vi "Theil-Sen.vi"(5 "Aligning array sizes? (T)":bool=TRUE, 6 "error in (no error)":errorcluster, 7 "Sen parameter":enum16{"Auto", "On", "Off"}(ring), 8 "input_Y":dbl[](array[numeric]), 9 "input_X":dbl[](array[numeric])) -> (0 "error out":errorcluster, 1 "b":dbl format="%.6g", 2 "m":dbl format="%.6g", 3 "output_Y":dbl[](array[numeric]))   [LabVIEW 2010]
doc: "The Theil–Sen estimator of a set of two-dimensional points (xi, yi) is the median m of the slopes (yj - yi)/(xj - xi) determined by all pairs of sample points. Sen extended this definition to handle the case in which two data points have the same x coordinate. In Sen's definition, one takes the median of the slopes defined only from pairs of points having distinct x coordinates.\nOnce the slope m has been determined, one may determine a line from the sample points by setting the y-intercept b to be the median of the values yi - mxi. The fit line is then the line y = mx + b with coefficients m and b in slope–intercept form."
uses:
  <vilib>/Analysis/NI_AALBase.lvlib
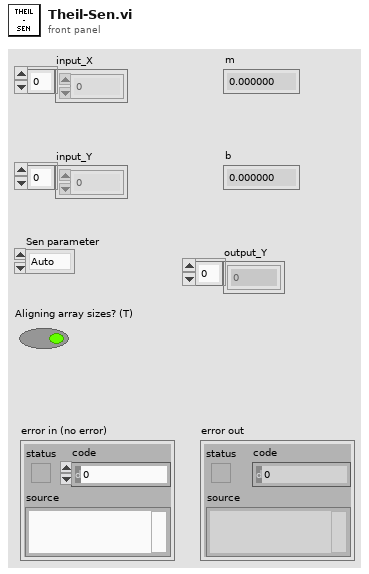
[diagram p1: front panel]
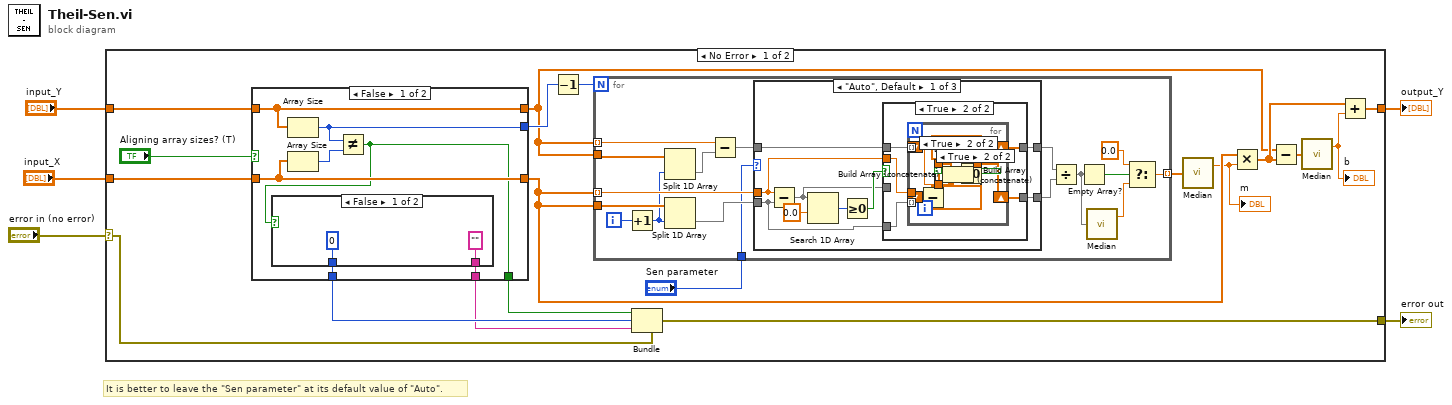
[diagram p0: block diagram]
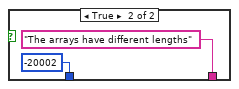
[diagram p2: hidden frame]
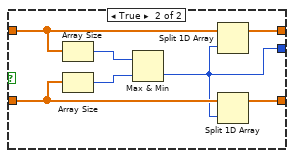
[diagram p3: hidden frame]
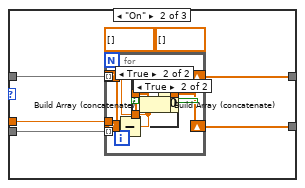
[diagram p7: hidden frame]
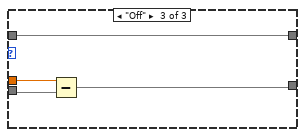
[diagram p10: hidden frame]
diagram:
  # "It is better to leave the \"Sen parameter\" at its default value of \"Auto\"."
  n1 = case shown="No Error" "error in (no error)" {
    selector: "error in (no error)" -> [w10 w124]
    tunnel: "input_X" -> [w24 _]
    tunnel: "input_Y" -> [w22 w123]
    tunnel: [w13 w124] -> w3
    tunnel: [w9 w123] -> w1
    frame No Error {
      n2 = case shown="False" "Aligning array sizes? (T)" {
        tunnel: w24 -> [w31 w40]
        tunnel: [w31 w39] -> w23
        tunnel: w22 -> [w30 w38]
        tunnel: [w30 w37] -> w7
        tunnel: [w26 _] -> w14
        tunnel: [w28 _] -> w12
        tunnel: [w27 _] -> w11
        tunnel: [w25 w36] -> w8
        frame False {
          n3 = Array Size(array=w30) -> (size(s)=w25:i32)
          n4 = Array Size(array=w31) -> (size(s)=w29:i32)
          n5 = Not Equal?(x=w25, y=w29) -> (x != y?=w26:bool)
          n6 = case shown="False" w26 {
            tunnel: [0 -20002] -> w28
            tunnel: ["" "The arrays have different lengths"] -> w27
            frame False {
            }
            frame True {
            }
          }
        }
        frame True {
          n7 = Array Size(array=w38) -> (size(s)=w42:i32)
          n8 = Array Size(array=w40) -> (size(s)=w41:i32)
          n9 = Max & Min(x=w42, y=w41) -> (min(x,y)=w36:i32)  [unwired: 1 out]
          n10 = Split 1D Array(array=w38, index=w36) -> (first subarray=w37:dbl[])  [unwired: 1 out]
          n11 = Split 1D Array(array=w40, index=w36) -> (first subarray=w39:dbl[])  [unwired: 1 out]
        }
      }
      n12 = Decrement(x=w8) -> (x-1=w21:i32)
      n13 = for {
        N: w21 -> [_]
        tunnel: w23 -> [w57] mode=indexing
        tunnel: w7 -> [w58]
        tunnel: w23 -> [w59]
        tunnel: [w45] -> w20 mode=indexing
        tunnel: w7 -> [w49] mode=indexing
        tunnel: "Sen parameter" -> [w48]
        i -> [w54]
        n14 = Increment(x=w54) -> (x+1=w53:i32)
        n15 = Split 1D Array(array=w58, index=w53) -> (second subarray=w55:dbl[])  [unwired: 1 out]
        n16 = Split 1D Array(array=w59, index=w53) -> (second subarray=w56:dbl[])  [unwired: 1 out]
        n17 = Subtract(x=w49, y=w55) -> (x-y=w51:dbl[])
        n18 = case shown="\"Auto\", Default" w48 {
          tunnel: w57 -> [w62 w101 w121]
          tunnel: w56 -> [w61 w100 w120]
          tunnel: [w67 w99 w119] -> w52
          tunnel: w51 -> [w66 w98 w122]
          tunnel: [w68 w97 w122] -> w50
          frame "Auto", Default {
            n19 = Subtract(x=w62, y=w61) -> (x-y=w60:dbl[])
            n20 = Search 1D Array(1D array=w60, element=0.0) -> (index of element=w64:i32)  [unwired: 1 in]
            n21 = Greater Or Equal To 0?(x=w64) -> (x >= 0?=w63:bool)
            n22 = case shown="True" w63 {
              tunnel: [w70 w77] -> w68
              tunnel: [w69 w76] -> w67
              tunnel: w66 -> [w70 w75]
              tunnel: w62 -> [_ w74]
              tunnel: w61 -> [_ w73]
              tunnel: w60 -> [w69 _]
              frame False {
              }
              frame True {
                n23 = for {
                  tunnel: w74 -> [w86]
                  tunnel: w73 -> [w85] mode=indexing
                  tunnel: w75 -> [w84] mode=indexing
                  shift-right: [w80] -> w76
                  shift-left: dbl[] [] ("Array") -> [w81]
                  shift-right: [w78] -> w77
                  shift-left: dbl[] [] ("Array") -> [w79]
                  n24 = Subtract(x=w86, y=w85) -> (x-y=w82:dbl)
                  n25 = Not Equal To 0?(x=w82) -> (x != 0?=w83:bool)
                  n26 = case shown="True" w83 {
                    tunnel: w79 -> [w87 w89]
                    tunnel: w84 -> [_ w88]
                    tunnel: [w87 w90] -> w78
                    frame False {
                    }
                    frame True {
                      n27 = Build Array (concatenate)(w89, w88) -> (w90:dbl[])
                    }
                  }
                  n28 = case shown="True" w83 {
                    tunnel: w81 -> [w91 w93]
                    tunnel: w82 -> [_ w92]
                    tunnel: [w91 w94] -> w80
                    frame False {
                    }
                    frame True {
                      n29 = Build Array (concatenate)(w93, w92) -> (w94:dbl[])
                    }
                  }
                }
              }
            }
          }
          frame "On" {
            n30 = for {
              tunnel: w101 -> [w110]
              tunnel: w100 -> [w109] mode=indexing
              tunnel: w98 -> [w108] mode=indexing
              shift-right: [w104] -> w99
              shift-left: dbl[] [] ("Array") -> [w105]
              shift-right: [w102] -> w97
              shift-left: dbl[] [] ("Array") -> [w103]
              n31 = Subtract(x=w110, y=w109) -> (x-y=w106:dbl)
              n32 = Not Equal To 0?(x=w106) -> (x != 0?=w107:bool)
              n33 = case shown="True" w107 {
                tunnel: w103 -> [w111 w113]
                tunnel: w108 -> [_ w112]
                tunnel: [w111 w114] -> w102
                frame False {
                }
                frame True {
                  n34 = Build Array (concatenate)(w113, w112) -> (w114:dbl[])
                }
              }
              n35 = case shown="True" w107 {
                tunnel: w105 -> [w115 w117]
                tunnel: w106 -> [_ w116]
                tunnel: [w115 w118] -> w104
                frame False {
                }
                frame True {
                  n36 = Build Array (concatenate)(w117, w116) -> (w118:dbl[])
                }
              }
            }
          }
          frame "Off" {
            n37 = Subtract(x=w121, y=w120) -> (x-y=w119:dbl[])
          }
        }
        n38 = Divide(x=w50, y=w52) -> (x/y=w46:dbl[])
        n39 = Empty Array?(array=w46) -> (empty?=w47:bool)
        n40 = call <vilib>:"Median.vi"("X"=w46) -> ("median"=w44:dbl)  [unwired: 1 out]
        n41 = Select(t=0.0, s=w47, f=w44) -> (s? t:f=w45:dbl)
      }
      n42 = Bundle(cluster=w10, "status"=w14, "code"=w12, "source"=w11) -> (w13:errorcluster)
      n43 = call <vilib>:"Median.vi"("X"=w20) -> ("median"=w17:dbl)  [unwired: 1 out]
      "m" <- w17
      n44 = Multiply(x=w23, y=w17) -> (x*y=w18:dbl[])
      n45 = Subtract(x=w7, y=w18) -> (x-y=w19:dbl[])
      n46 = call <vilib>:"Median.vi"("X"=w19) -> ("median"=w16:dbl)  [unwired: 1 out]
      "b" <- w16
      n47 = Add(x=w18, y=w16) -> (x+y=w9:dbl[])
    }
    frame Error {
    }
  }
  "error out" <- w3
  "output_Y" <- w1
